vi "Write DAC.vi"(8 "error in (no error)":errorcluster, 9 "Analog Output V1":u16, 10 "Analog Output VO":u16, 11 "M5StackDAC2 in":refnum<class "M5StackDAC2.lvclass">) -> (0 "error out":errorcluster, 3 "M5StackDAC2 out":refnum<class "M5StackDAC2.lvclass">)   [LabVIEW 2020, in "CTI-Peripheral.lvlib" / "M5StackDAC2.lvclass"]
uses:
  M5StackDAC2.lvclass
  M5StackDAC2.lvclass/M5StackDAC2.ctl
  CTI/I2C Connection/I2C Connection.lvclass/I2C Connection.ctl
  CTI/I2C Connection/I2C Connection.lvclass
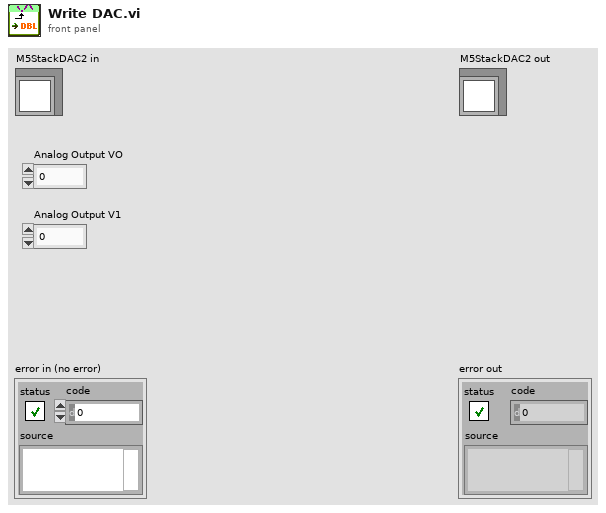
[diagram p1: front panel]
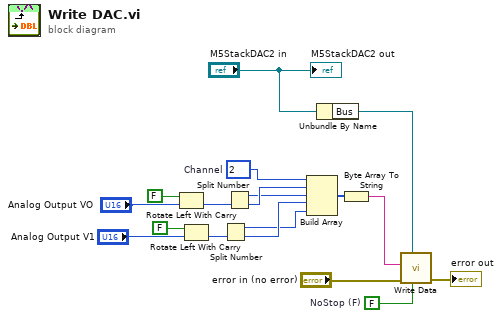
[diagram p0: block diagram]
diagram:
  w14 = u8 2  # Channel
  w15 = FALSE  # NoStop (F)
  n1 = Rotate Left With Carry(2:"Analog Output VO", 3:FALSE ("carry")) -> (0:w12:u16)  [unwired: 1 out]
  n2 = Rotate Left With Carry(2:"Analog Output V1", 3:FALSE ("carry")) -> (0:w10:u16)  [unwired: 1 out]
  n3 = Split Number(x=w10) -> (hi(x)=w6:u8, lo(x)=w7:u8)
  n4 = Split Number(x=w12) -> (hi(x)=w8:u8, lo(x)=w9:u8)
  n5 = Build Array(w14, w9, w8, w7, w6) -> (w5:u8[])
  n6 = Unbundle By Name("M5StackDAC2 in") -> ("Bus"=w16:refnum<class "I2C Connection.lvclass">)
  n7 = Byte Array To String(unsigned byte array=w5) -> (string=w2:string)
  n8 = call "Write Data.vi"("NoStop (F)"=w15, "I2C Connection"=w16, "error in (no error)"="error in (no error)", "Data"=w2) -> ("error out"=→"error out":errorcluster)  [unwired: 7 in]
  "M5StackDAC2 out" <- "M5StackDAC2 in"
